vi "Remove Methods.vi"(8 "error in (no error)":errorcluster, 10 "Methods":string[](array[string]), 11 "LUnit Test Suite V2 in":refnum<class "LUnit Test Suite V2.lvclass">) -> (0 "error out":errorcluster, 3 "LUnit Test Suite V2 out":refnum<class "LUnit Test Suite V2.lvclass">)   [LabVIEW 2020, in "LUnit Test Suite V2.lvclass"]
uses:
  LUnit Test Suite V2.lvclass
  LUnit Test Suite V2.lvclass/LUnit Test Suite V2.ctl
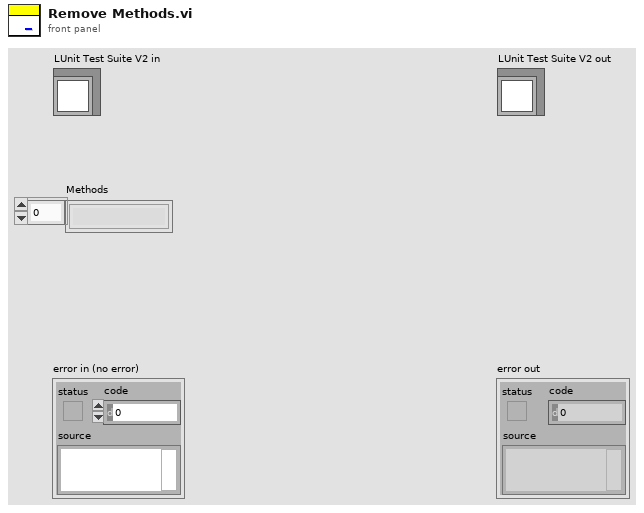
[diagram p1: front panel]
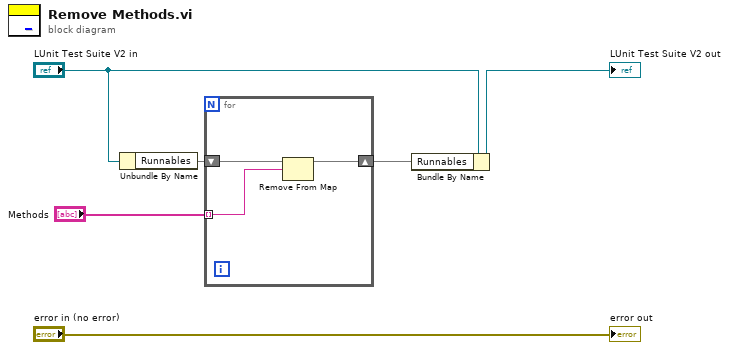
[diagram p0: block diagram]
diagram:
  n1 = Unbundle By Name("LUnit Test Suite V2 in") -> ("Runnables"=w4:map{string, refnum<class "Runnable.lvclass">})
  n2 = for {
    shift-right: [w7] -> w2
    shift-left: w4 -> [w8]
    tunnel: "Methods" -> [w9] mode=indexing
    n3 = Remove From Map(10:w9, 11:w8) -> (3:w7:map{string, refnum<class "Runnable.lvclass">})  [unwired: 2 out]
  }
  n4 = Bundle By Name(cluster="LUnit Test Suite V2 in", "Runnables"=w2) -> (→"LUnit Test Suite V2 out":refnum<class "LUnit Test Suite V2.lvclass">)
  "error out" <- "error in (no error)"
